vi "Write To Connection.vi"(8 "error in (no error)":errorcluster, 10 "Data to Write":string, 11 "ProtectedConnectionWriter in":refnum<class "ProtectedConnectionWriter.lvclass">) -> (0 "error out":errorcluster)   [LabVIEW 2019, in "ProtectedConnectionWriter.lvclass"]
uses:
  <vilib>/gpm_packages/@cs/Network-interface/Source/ProtectedConnectionWriter/ProtectedConnectionWriter.lvclass
  <vilib>/gpm_packages/@cs/Network-interface/Source/ProtectedConnectionWriter/ProtectedConnectionWriter.lvclass/ProtectedConnectionWriter.ctl
  <vilib>/gpm_packages/@cs/Network-interface/Source/Connection Reference/Connection Reference/Connection Reference.lvclass/Connection Reference.ctl
  <vilib>/gpm_packages/@cs/Network-interface/Source/Connection Reference/IConnection/IConnection.lvclass
  <vilib>/gpm_packages/@cs/Network-interface/Source/Connection Reference/Connection Reference/Connection Reference.lvclass
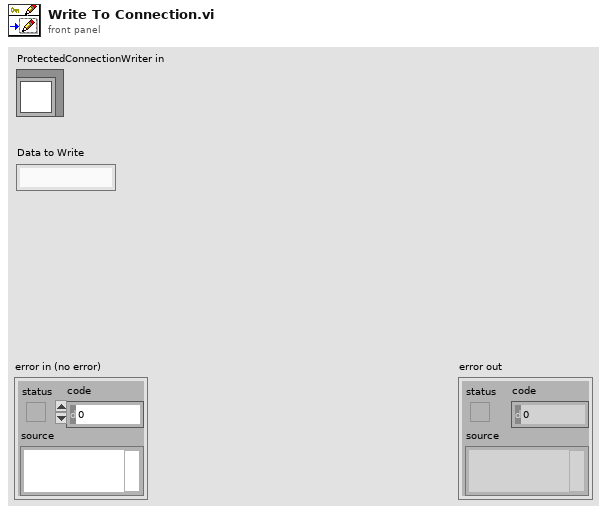
[diagram p1: front panel]
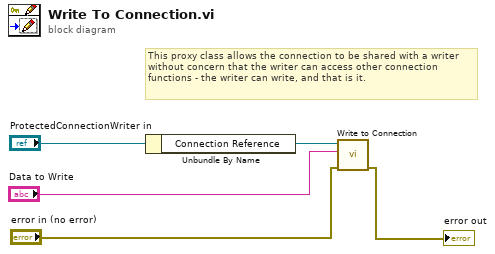
[diagram p0: block diagram]
diagram:
  # "This proxy class allows the connection to be shared with a writer without concern that the writer can access other connection functions - the writer can write, and that is it."
  n1 = Unbundle By Name("ProtectedConnectionWriter in") -> ("Connection Reference"=w4:refnum<data-value>)
  n2 = call <vilib>:"Write to Connection.vi"("error in (no error)"="error in (no error)", "Data to Write"="Data to Write", "Connection Reference In"=w4) -> ("error out"=→"error out":errorcluster)  [unwired: 7 in, 1 out]
